vi "test to disable enum values.vi"() -> ()   [LabVIEW 2021]
uses:
  type-defs/odor selection (type def).ctl
  a3a82ab2-025a-4ef7-b04c-7f4889cd4c6b.vi
panel:
  in  "odor selection 2":T1
  in  "Stop":bool
  in  "error in (no error)":errorcluster
  out "error out":errorcluster
  in  "Remove Odd Odors":bool
  in  "odor selection":T1
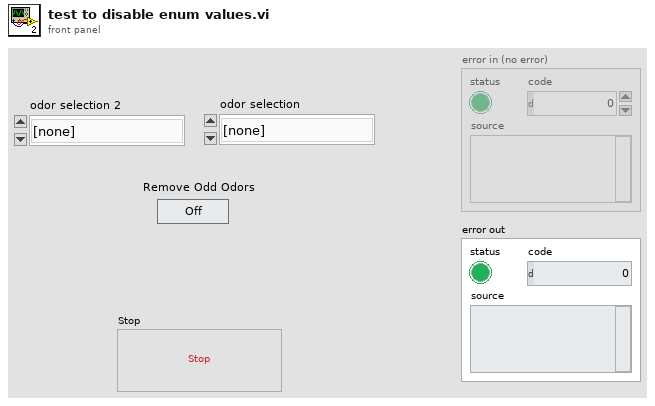
[diagram p1: front panel]
types:
  T1 = typedef "odor selection (type def).ctl" = enum16{"[none]", "odor 1", "odor 2", "odor 3", "odor 4", "odor 5", "odor 6", "odor 7", "odor 8", "odor 9", "odor 10"}
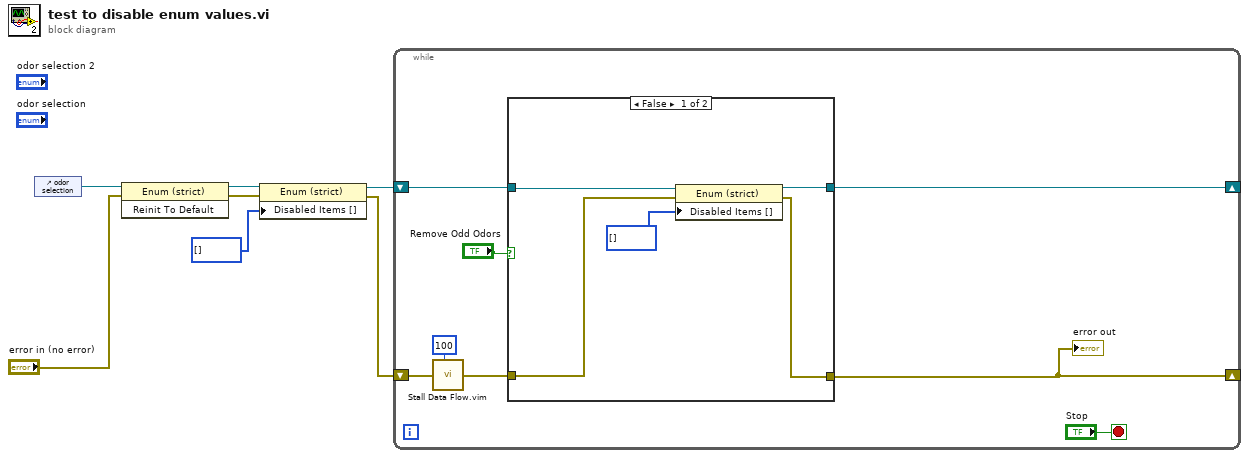
[diagram p0: block diagram]
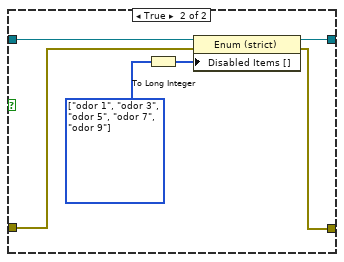
[diagram p2: hidden frame]
diagram:
  n1 = control-ref of="odor selection"() -> (w6:refnum<vi>)
  n2 = invoke class="Enum (strict)" method="Reinit To Default"(reference=w6, error in="error in (no error)") -> (reference out=w3:refnum<vi>, error out=w5:errorcluster)  [unwired: 1 in, 1 out]
  n3 = property class="Enum (strict)"(reference=w3, error in=w5, "Disabled Items []"=i32[] []) -> (reference out=w2:refnum<vi>, error out=w4:errorcluster)
  n4 = while {
    shift-right: [w11] -> _
    shift-left: w4 -> [w12]
    shift-right: [w13] -> _
    shift-left: w2 -> [w15]
    stop <- "Stop" stop-if-true
    n5 = call "Stall Data Flow.vim"("value in"=w12, "milliseconds to wait"=u32 100) -> ("value out"=w9:errorcluster)  [unwired: 1 out]
    n6 = case shown="False" "Remove Odd Odors" {
      tunnel: w15 -> [w16 w26]
      tunnel: [w19 w22] -> w13
      tunnel: w9 -> [w17 w25]
      tunnel: [w18 w21] -> w11
      frame False {
        n7 = property class="Enum (strict)"(reference=w16, error in=w17, "Disabled Items []"=i32[] []) -> (reference out=w19:refnum<vi>, error out=w18:errorcluster)
      }
      frame True {
        w24 = T1[] [enum."odor 1", enum."odor 3", enum."odor 5", enum."odor 7", enum."odor 9"] items=["[none]", "odor 1", "odor 2", "odor 3", "odor 4", "odor 5", "odor 6", "odor 7", "odor 8", "odor 9", "odor 10"] ("Disabled Items []")
        n8 = To Long Integer(number=w24) -> (32bit integer=w23:i32[])
        n9 = property class="Enum (strict)"(reference=w26, error in=w25, "Disabled Items []"=w23) -> (reference out=w22:refnum<vi>, error out=w21:errorcluster)
      }
    }
    "error out" <- w11
  }
